vi "计算行列号.vi"(8 "垂直偏移":i16, 9 "水平偏移":i16, 10 "垂直":i16, 11 "水平":i16) -> (2 "列":i16, 3 "行":i16)   [LabVIEW 2012]
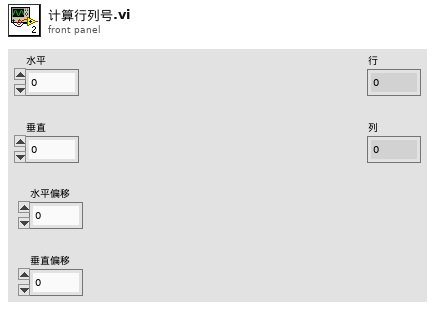
[diagram p1: front panel]
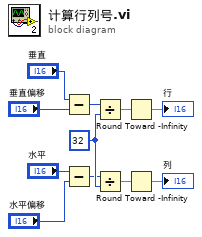
[diagram p0: block diagram]
diagram:
  w7 = 32
  n1 = Subtract(x="垂直", y="垂直偏移") -> (x-y=w5:i16)
  n2 = Subtract(x="水平", y="水平偏移") -> (x-y=w3:i16)
  n3 = Divide(x=w5, y=w7) -> (x/y=w10:dbl)
  n4 = Divide(x=w3, y=w7) -> (x/y=w11:dbl)
  n5 = Round Toward -Infinity(1:w10) -> (0:→"行":dbl)
  n6 = Round Toward -Infinity(1:w11) -> (0:→"列":dbl)
